vi "Get UI Vals.vi"(11 "Series UI Actor in":refnum<class "Series UI Actor.lvclass">) -> (2 "UI Vals":map{string, cluster{"New?":bool, variant}}(c390), 3 "Series UI Actor out":refnum<class "Series UI Actor.lvclass">)   [LabVIEW 2024, in "Series UI Actor.lvlib" / "Series UI Actor.lvclass"]
uses:
  Series UI Actor.lvclass
  Series UI Actor.lvclass/Series UI Actor.ctl
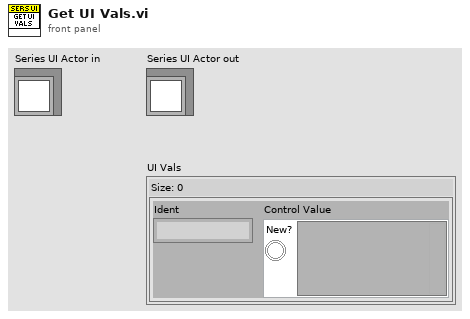
[diagram p1: front panel]
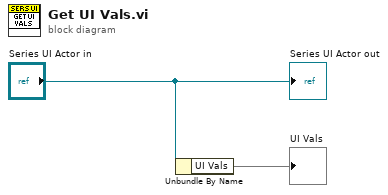
[diagram p0: block diagram]
diagram:
  n1 = Unbundle By Name("Series UI Actor in") -> ("UI Vals"=→"UI Vals":map{string, cluster{"New?":bool, variant}})
  "Series UI Actor out" <- "Series UI Actor in"
